vi "Main.vi"() -> ()   [LabVIEW 2018]
uses:
  <vilib>/myRIO/Instrument Drivers/Onboard IO/I2C/typedefs/I2C User Configuration.ctl
  <vilib>/myRIO/Instrument Drivers/Onboard IO/I2C/typedefs/I2C Transfer Rate.ctl
  <vilib>/Platform/TimedLoop/XDataNode/timing_clust.ctl
  <vilib>/Platform/TimedLoop/XDataNode/nitl_modes.ctl
  <vilib>/Platform/TimedLoop/XDataNode/wakeup.ctl
  <vilib>/myRIO/Common/Instrument Driver Framework/myRIO v1.0/DIO/vis/myRIO v1.1 Open DIO.vi
  <vilib>/myRIO/Common/Instrument Driver Framework/myRIO v1.0/I2C/vis/myRIO v1.1 Open I2C.vi
  <vilib>/myRIO/Common/Instrument Driver Framework/myRIO v1.0/UART/vis/myRIO v1.0 Close UART.vi
  <vilib>/myRIO/Common/Instrument Driver Framework/Utilities/vis/Validate Channels.vi
  <vilib>/myRIO/Common/Instrument Driver Framework/myRIO v1.0/DIO/vis/myRIO v1.0 Reserve DIO.vi
  <vilib>/myRIO/Common/Instrument Driver Framework/myRIO v1.0/I2C/vis/myRIO v1.0 Reserve I2C.vi
  <vilib>/myRIO/Common/Instrument Driver Framework/myRIO v1.0/Resource Manager/vis/myRIO v1.0 Reserve Channel List.vi
  <vilib>/myRIO/Common/Instrument Driver Framework/myRIO v1.0/DIO/vis/myRIO v1.0 Build MUX Configuration DIO.vi
  <vilib>/myRIO/Common/Instrument Driver Framework/myRIO v1.0/I2C/vis/myRIO v1.0 Build MUX Configuration I2C.vi
  <vilib>/myRIO/Common/Instrument Driver Framework/myRIO v1.0/Resource Manager/vis/myRIO v1.0 Reserve Channel.vi
  <vilib>/myRIO/Common/Instrument Driver Framework/myRIO v1.0/Resource Manager/vis/myRIO v1.0 Unreserve Channel.vi
  <vilib>/myRIO/Common/Instrument Driver Framework/myRIO v1.0/Resource Manager/vis/myRIO v1.0 Create Configuration List.vi
  <vilib>/myRIO/Common/Instrument Driver Framework/myRIO v1.0/Resource Manager/vis/myRIO v1.0 Build Mutex Name.vi
  <vilib>/Utility/VariantDataType/GetNumericInfo.vi
  <vilib>/Utility/error.llb/Error Cluster From Error Code.vi
  <vilib>/myRIO/Common/Instrument Driver Framework/myRIO v1.0/myRIO v1.1 Open.vi
  <vilib>/myRIO/Common/Instrument Driver Framework/Utilities/vis/IO Manager.vi
  <vilib>/myRIO/Common/Instrument Driver Framework/Utilities/vis/Configuration Manager.vi
  <vilib>/myRIO/Common/Instrument Driver Framework/myRIO v1.0/Resource Manager/vis/myRIO v1.0 Configure IO.vi
  <vilib>/myRIO/Common/Instrument Driver Framework/myRIO v1.0/myRIO v1.0 Close.vi
  <vilib>/myRIO/Common/Instrument Driver Framework/myRIO v1.0/I2C/vis/myRIO v1.0 Configure I2C.vi
  <vilib>/myRIO/Common/Instrument Driver Framework/myRIO v1.0/I2C/vis/myRIO v1.0 Write I2C.vi
  <vilib>/myRIO/Common/Instrument Driver Framework/myRIO v1.0/DIO/vis/myRIO v1.0 Read DIO.vi
  <vilib>/myRIO/Common/Instrument Driver Framework/myRIO v1.0/DIO/vis/myRIO v1.0 Write DIO.vi
  <vilib>/myRIO/Common/Instrument Driver Framework/myRIO v1.0/I2C/vis/myRIO v1.0 Read I2C.vi
  <vilib>/myRIO/Common/Instrument Driver Framework/Utilities/vis/FPGA Ref Manager.vi
  <vilib>/myRIO/Common/Instrument Driver Framework/myRIO v1.0/myRIO v1.0 Reset FPGA.vi
  <vilib>/myRIO/Common/Instrument Driver Framework/myRIO v1.0/IRQ/vis/myRIO v1.0 IRQ Info FGV.vi
  <vilib>/myRIO/Common/Instrument Driver Framework/myRIO v1.0/IRQ/vis/myRIO v1.0 Timer IRQ Info FGV.vi
  <vilib>/myRIO/Common/Instrument Driver Framework/myRIO v1.0/IRQ/vis/myRIO v1.0 ISR Agent.vi
  <vilib>/Platform/TimedLoop/XDataNode/XDataNode.xnode
  <vilib>/myRIO/Instrument Drivers/Utilities/Utilities.lvlib
  <vilib>/myRIO/Instrument Drivers/Onboard IO/I2C/I2C.lvlib
  <vilib>/myRIO/Instrument Drivers/Onboard IO/DIO/DIO.lvlib
  <vilib>/Platform/TimedLoop/XDataNode/XDNodeRunTimeDep.lvlib
panel:
  out "arccos(x)":dbl
  out "배열":errorcluster[](array[cluster])
  out "INT_SOURCE":bool[](array[boolean])
  out "Waveform Chart":cluster{i16, i16, i16}(graph)
  out "DATA":u8[](array[numeric]) format="%02x"
  out "Z":i16
  out "Y":i16
  out "X":i16
  in  "[ESC]":bool
  # "Accelerometer demo"
  # "DATAX0"
  # "DATAX1"
  # "DATAY0"
  # "DATAY1"
  # "DATAZ0"
  # "DATAZ1"
  # "D = data ready\n1T = single-tap\n2T = double-tap"
  # "A = activity\nI = inactivity\nF = free fall"
  # "W = watermark\nO = overrun"
  # "D   1T  2T   A    I     F    W   O"
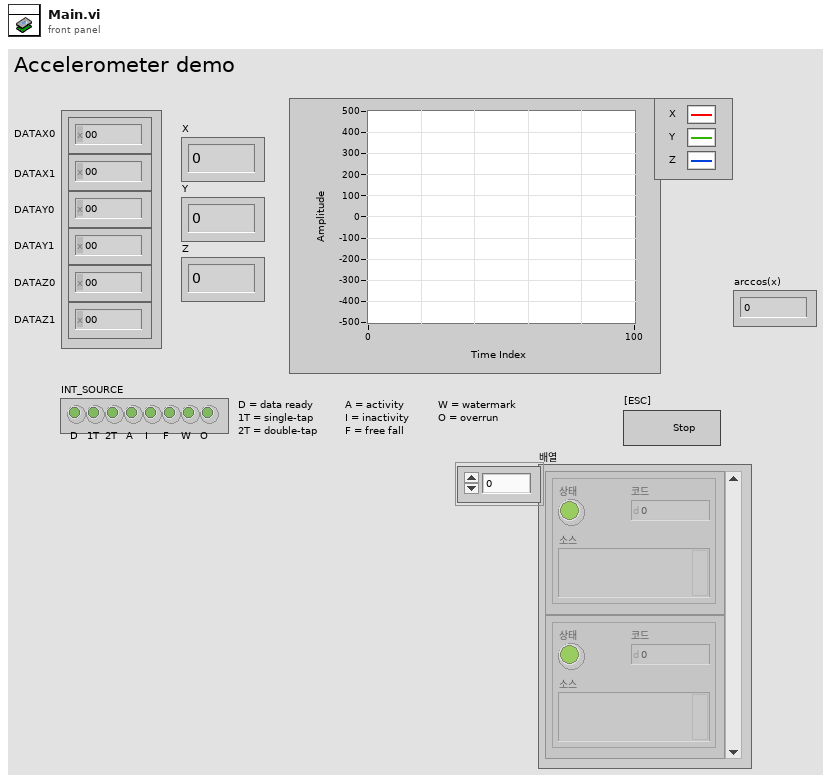
[diagram p1: front panel]
types:
  T1 = typedef "I2C.lvlib/I2C User Configuration.ctl" = cluster{"I2C Transfer Rate":T2}
  T2 = typedef "I2C.lvlib/I2C Transfer Rate.ctl" = enum16{"Standard mode (100 kbps)", "Fast mode (400 kbps)"}
  T3 = typedef "I2C.lvlib/I2C Reference.ctl" = cluster{"myRIO Reference":T4, "I2C Channels Enum":T8, "I2C Configuration":T9}
  T4 = typedef "myRIO Generic Hardware Reference.ctl" = cluster{"myRIO Model":T5, "myRIO Hardware Reference":T6}
  T5 = typedef "Hardware Version Enum.ctl" = enum16{"Unknown", "myRIO-1900", "myRIO-1950", "roboRIO", "NI ELVIS RIO CM", "ELVIS III"}
  T6 = typedef "myRIO v1.0 Reference.ctl" = cluster{"Generic FPGA Reference":T7, "Allow multiple opens":bool}
  T7 = typedef "Generic FPGA Reference.ctl" = refnum<k20>
  T8 = typedef "I2C Channels Enum.ctl" = enum16{"Not Connected", "A/I2C", "B/I2C", "I2C/I2C"}
  T9 = typedef "I2C.lvlib/I2C Configuration.ctl" = cluster{"I2C Transfer Rate":T2}
  T10 = typedef "DIO.lvlib/DIO Reference.ctl" = cluster{"myRIO Reference":T4, "DIO Channels List":T11}
  T11 = typedef "DIO Channels List.ctl" = T12[]
  T12 = typedef "DIO Channels Enum.ctl" = enum16{"Not Connected", "C/DIO0", "C/DIO1", "C/DIO2", "C/DIO3", "C/DIO4", "C/DIO5", "C/DIO6", "C/DIO7", "A/DIO0", "A/DIO1", "A/DIO2", "A/DIO3", "A/DIO4", "A/DIO5", "A/DIO6", "A/DIO7", "A/DIO8", "A/DIO9", "A/DIO10", "A/DIO11", "A/DIO12", "A/DIO13", "A/DIO14", "A/DIO15", "A/DIO16", "A/DIO17", "A/DIO18", "A/DIO19", "B/DIO0", "B/DIO1", "B/DIO2", "B/DIO3", "B/DIO4", "B/DIO5", "B/DIO6", "B/DIO7", "B/DIO8", "B/DIO9", "B/DIO10", "B/DIO11", "B/DIO12", "B/DIO13", "B/DIO14", "B/DIO15", "B/DIO16", "B/DIO17", "B/DIO18", "B/DIO19", "LED0", "LED1", "LED2", "LED3", "Button0", "DIO/DIO0", "DIO/DIO1", "DIO/DIO2", "DIO/DIO3", "DIO/DIO4", "DIO/DIO5", "DIO/DIO6", "DIO/DIO7", "DIO/DIO8", "DIO/DIO9", "SPI/CS0", "SPI/CS1", "SPI/CS2", "SPI/CS3", "LED RADIO (Green)", "LED RADIO (Red)", "LED COMM (Green)", "LED COMM (Red)", "LED MODE (Green)", "LED MODE (Red)"}
  T13 = typedef "XDNodeRunTimeDep.lvlib/timing_clust.ctl" = cluster{"Expected End [f-1]":u64, "Actual End [f-1]":u64, "Finished Late? [f-1]":bool, "Expected End [i-1]":u64, "Actual End [i-1]":u64, "Finished Late? [i-1]":bool, "Expected Start [i]":u64, "Actual Start [i]":u64, "Expected Start [f]":u64, "Actual Start [f]":u64, "Source Name":string, "Structure Name":string, "Period":i64, "Deadline":i64, "Offset":i64, "Start":i64, "Priority":i32, "Timeout":i32, "Mode":T14, "Wakeup Reason":T15, "Error":errorcluster, "Source Type":string, "Secondary Source Type":string, "Global End Time":u64, "Global Start Time":u64, "Frame Duration":u64, "Iteration Duration":u64, "Assigned CPU":i32, "I/O Scan Engine Mode":u32}
  T14 = typedef "XDNodeRunTimeDep.lvlib/nitl_modes.ctl" = enum32{"No Change", "Process missed periods, maintain original phase", "Discard missed periods, maintain original phase", "Process missed periods, ignore original phase", "Discard missed periods, ignore original phase"}
  T15 = typedef "XDNodeRunTimeDep.lvlib/wakeup.ctl" = enum32{"Normal", "Aborted", "Asynchronous wakeup", "Timing source error", "Timed loop error", "Timeout"}
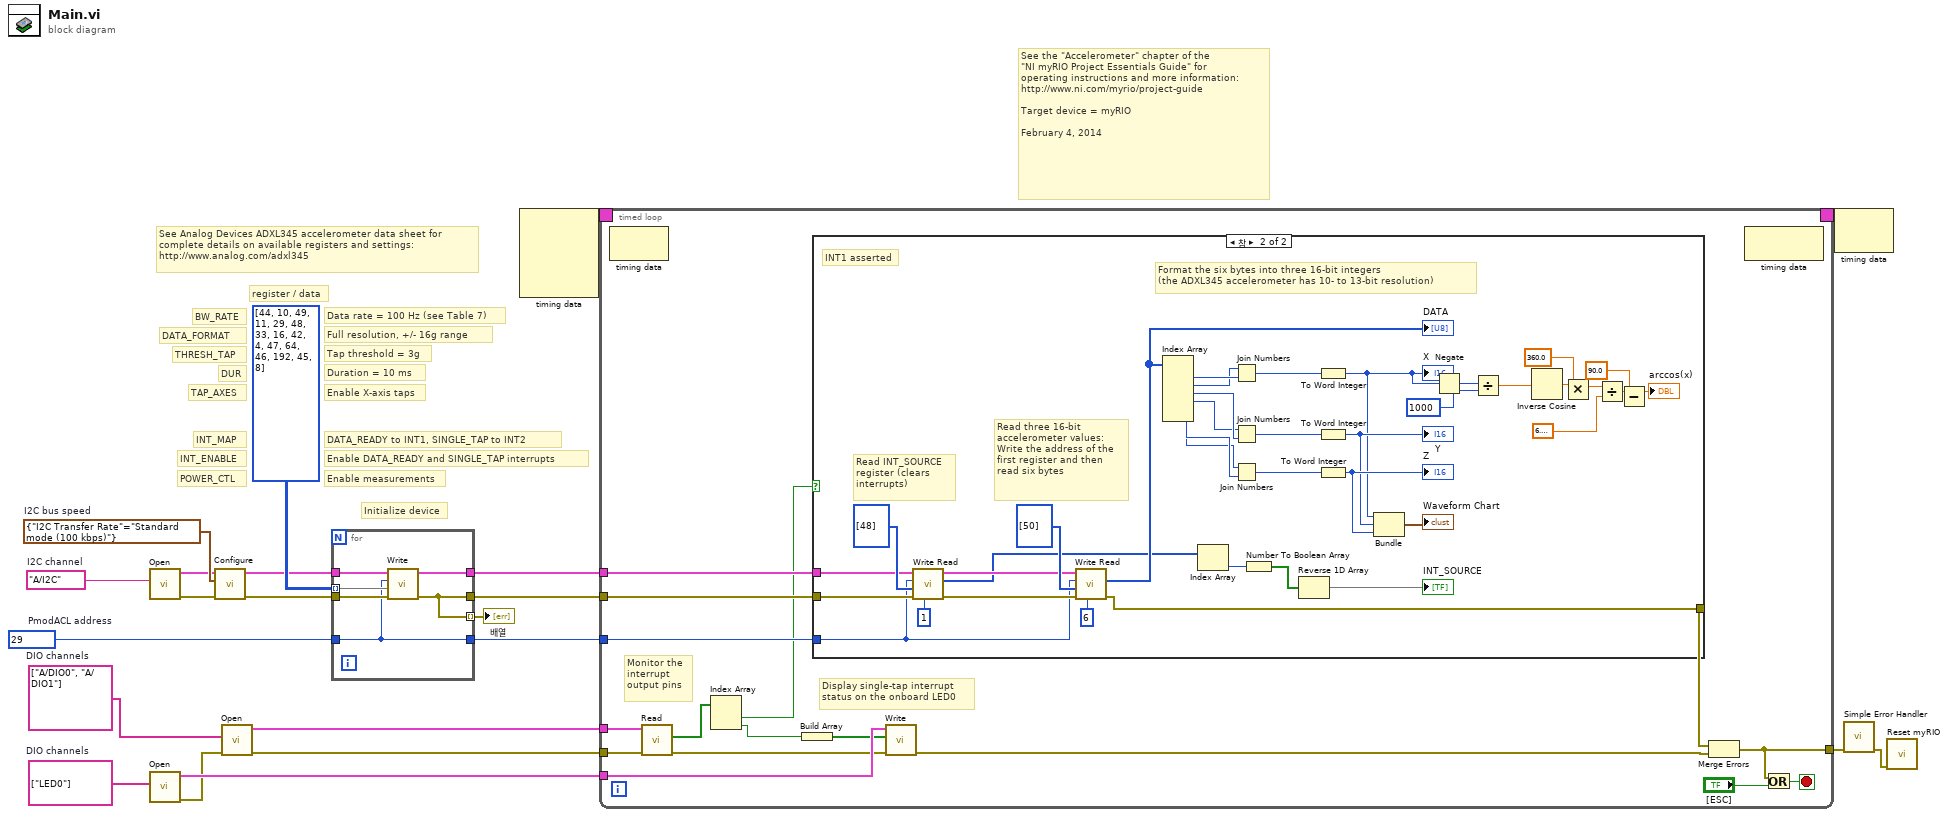
[diagram p0: block diagram]
diagram:
  w4 = tag[] ["LED0"]  # DIO channels
  w7 = tag[] ["A/DIO0", "A/DIO1"]  # DIO channels
  w19 = T1 {"I2C Transfer Rate"=enum."Standard mode (100 kbps)"}  # I2C bus speed
  w20 = tag "A/I2C"  # I2C channel
  w10 = u8 29  # PmodACL address
  # "See the \"Accelerometer\" chapter of the\n\"NI myRIO Project Essentials Guide\" for\noperating instructions and more information: \nhttp://www.ni.com/myrio/project-guide\n\nTarget device = myRIO\n\nFebruary 4, 2014"
  # "Data rate = 100 Hz (see Table 7)"
  # "BW_RATE"
  # "DATA_READY to INT1, SINGLE_TAP to INT2"
  # "INT_MAP"
  # "Enable X-axis taps"
  # "TAP_AXES"
  # "Initialize device"
  # "Enable measurements"
  # "Enable DATA_READY and SINGLE_TAP interrupts"
  # "Duration = 10 ms"
  # "Tap threshold = 3g"
  # "See Analog Devices ADXL345 accelerometer data sheet for\ncomplete details on available registers and settings:\nhttp://www.analog.com/adxl345"
  # "POWER_CTL"
  # "INT_ENABLE"
  # "DUR"
  # "THRESH_TAP"
  # "Full resolution, +/- 16g range"
  # "DATA_FORMAT"
  # "register / data"
  n1 = call <vilib>:"Open.vi"("Channel Name"=w20) -> ("error out"=w17:errorcluster, "I2C Ref Out"=w18:T3)  [unwired: 9 in]
  n2 = call <vilib>:"Open.vi"("Channel Names"=w4) -> ("error out"=w2:errorcluster, "DIO Ref Out"=w3:T10)  [unwired: 9 in]
  n3 = call <vilib>:"Configure.vi"("error in (no error)"=w17, "I2C User Configuration"=w19, "I2C Ref In"=w18) -> ("error out"=w11:errorcluster, "I2C Ref Out"=w12:T3)  [unwired: 7 in]
  n4 = call <vilib>:"Open.vi"("error in (no error)"=w2, "Channel Names"=w7) -> ("error out"=w9:errorcluster, "DIO Ref Out"=w8:T10)  [unwired: 8 in]
  n5 = for {
    tunnel: [w23] -> w16
    tunnel: [w28] -> w15
    tunnel: [w24] -> w14
    tunnel: u8[][] [[44, 10], [49, 11], [29, 48], [33, 16], [42, 4], [47, 64], [46, 192], [45, 8]] ("Bytes to Write") -> [w27] mode=indexing
    tunnel: w12 -> [w26]
    tunnel: w11 -> [w25]
    tunnel: w10 -> [w24]
    tunnel: [w23] -> w1 mode=indexing
    n6 = call <vilib>:"Write.vi"("error in (no error)"=w25, "Bytes to Write"=w27, "Slave Address (7-bit)"=w24, "I2C Ref In"=w26) -> ("error out"=w23:errorcluster, "I2C Ref Out"=w28:T3)  [unwired: 6 in]
  }
  "배열" <- w1
  n7 = node-c288() -> (w6:T13)  [unwired: 4 in]
  n8 = timed-loop {
    tunnel: [w29] -> w21
    tunnel: w14 -> [w40]
    tunnel: w16 -> [w42]
    tunnel: w15 -> [w41]
    tunnel: w9 -> [w39]
    tunnel: w8 -> [w38]
    timing: w6 -> [_]
    timing-out: [_] -> w5
    tunnel: w3 -> [w34]
    stop <- w44 stop-if-true
    # "Display single-tap interrupt\nstatus on the onboard LED0"
    # "Monitor the\ninterrupt\noutput pins"
    n9 = node-c288() -> ()  [unwired: 1 in, 1 out]
    n10 = call <vilib>:"Read.vi"("error in (no error)"=w39, "DIO Ref In"=w38) -> ("error out"=w33:errorcluster, "Values"=w35:bool[])  [unwired: 7 in, 1 out]
    n11 = Index Array "Index Array"(array=w35) -> (element #1=w36:bool, element #2=w31:bool)  [unwired: 2 in]
    n12 = Build Array "Build Array"(w31) -> (w32:bool[])
    n13 = case shown="참" w36 {
      tunnel: w42 -> [w47 w77]
      tunnel: w41 -> [_ w76]
      tunnel: w40 -> [_ w65]
      tunnel: [w47 w61] -> w37
      frame False {
        # "INT1 deasserted"
      }
      frame True {
        # "INT1 asserted"
        # "Read INT_SOURCE\nregister (clears\ninterrupts)"
        # "Read three 16-bit accelerometer values:\nWrite the address of the first register and then read six bytes"
        # "Format the six bytes into three 16-bit integers\n(the ADXL345 accelerometer has 10- to 13-bit resolution)"
        n14 = call <vilib>:"Write Read.vi"("Byte Count"=u32 1, "error in (no error)"=w77, "Bytes to Write"=u8[] [48], "Slave Address (7-bit)"=w65, "I2C Ref In"=w76) -> ("error out"=w66:errorcluster, "Bytes Read"=w59:u8[], "I2C Ref Out"=w67:T3)  [unwired: 3 in]
        n15 = call <vilib>:"Write Read.vi"("Byte Count"=u32 6, "error in (no error)"=w66, "Bytes to Write"=u8[] [50], "Slave Address (7-bit)"=w65, "I2C Ref In"=w67) -> ("error out"=w61:errorcluster, "Bytes Read"=w60:u8[])  [unwired: 3 in, 1 out]
        "DATA" <- w60
        n16 = Index Array "Index Array"(array=w60) -> (element #1=w75:u8, element #2=w74:u8, element #3=w73:u8, element #4=w72:u8, element #5=w71:u8, element #6=w70:u8)  [unwired: 6 in]
        n17 = Index Array "Index Array"(array=w59) -> (element=w64:u8)  [unwired: 1 in]
        n18 = Join Numbers(hi=w74, lo=w75) -> ((hi.lo)=w85:u16)
        n19 = Join Numbers(hi=w72, lo=w73) -> ((hi.lo)=w84:u16)
        n20 = Join Numbers(hi=w70, lo=w71) -> ((hi.lo)=w83:u16)
        n21 = Number To Boolean Array(number=w64) -> (Boolean array=w63:bool[])
        n22 = Reverse 1D Array(array=w63) -> (reversed array=→"INT_SOURCE":bool[])
        n23 = To Word Integer(number=w85) -> (16bit integer=w58:i16)
        "X" <- w58
        n24 = To Word Integer(number=w84) -> (16bit integer=w80:i16)
        "Y" <- w80
        n25 = To Word Integer(number=w83) -> (16bit integer=w82:i16)
        "Z" <- w82
        n26 = Bundle "Bundle"(w58, w80, w82) -> (→"Waveform Chart":cluster{i16, i16, i16})  [unwired: 1 in]
        n27 = Negate(x=w58) -> (-x=w50:i16)
        n28 = Divide(x=w50, y=i16 1000) -> (x/y=w56:dbl)
        n29 = Inverse Cosine(1:w56) -> (0:w55:dbl)
        n30 = Multiply(x=w55, y=360.0) -> (x*y=w54:dbl)
        n31 = Divide(x=w54, y=6.283185307179586) -> (x/y=w52:dbl)
        n32 = Subtract(x=w52, y=90.0) -> (x-y=→"arccos(x)":dbl)
      }
    }
    n33 = call <vilib>:"Write.vi"("error in (no error)"=w33, "Values"=w32, "DIO Ref In"=w34) -> ("error out"=w30:errorcluster)  [unwired: 6 in, 1 out]
    n34 = Merge Errors "Merge Errors"(w37, w30) -> (w29:errorcluster)
    n35 = node-c288() -> ()  [unwired: 1 in, 1 out]
    n36 = Or(x=w29, y="[ESC]") -> (x .or. y?=w44:bool)
  }
  n37 = node-c288(w5) -> ()  [unwired: 1 out]
  n38 = call <vilib>:"Simple Error Handler.vi"("error in (no error)"=w21) -> ("error out"=w22:errorcluster)  [unwired: 4 in, 4 out]
  n39 = call <vilib>:"Reset myRIO.vi"("error in (no error)"=w22) -> ()  [unwired: 10 in, 1 out]
